vi "Romi-Drive-System-Set-Speed-Demand.vi"(9 "Right Speed Demand":dbl, 11 "Left Speed Demand":dbl) -> ()   [LabVIEW 2019]
uses:
  Romi-Drive-System-Globals.vi
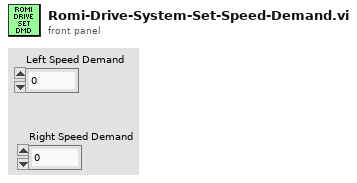
[diagram p1: front panel]
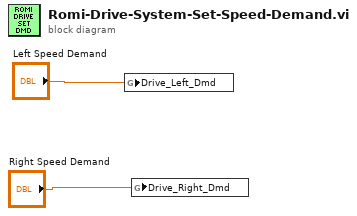
[diagram p0: block diagram]
diagram:
  n1 = global write "Romi-Drive-System-Globals.vi" "Drive_Left_Dmd"("Left Speed Demand") -> ()
  n2 = global write "Romi-Drive-System-Globals.vi" "Drive_Right_Dmd"("Right Speed Demand") -> ()
